vi "Volt2Photon.vi"() -> ()   [LabVIEW 2019]
panel:
  out "Actual Output (V)":dbl format="%#_6p"
  in  "Lockin Sensitivity":dbl format="%#_3p"
  in  "Lockin Output (V)":dbl format="%#_3p"
  out "Mean Power (W)":dbl=-4.8720373573303983e-11 format="%#.3p"
  out "Photons/Pulse":ext=-1.22632021926945247725 format="%#.4g"
  in  "Repetition Rate (Hz)":ext[unit]=80000000.0 format="%#_6p"
  in  "Wavelength (m)":dbl=4e-07 format="%#_6p"
  out "Photons/Second":ext[unit]=-98105617.54155619818 format="%#.0p"
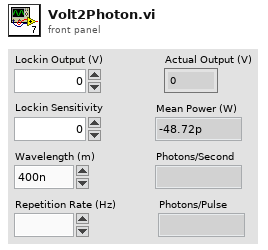
[diagram p1: front panel]
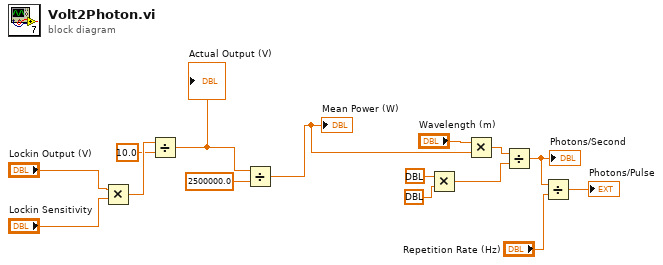
[diagram p0: block diagram]
diagram:
  n1 = Multiply(x="Lockin Output (V)", y="Lockin Sensitivity") -> (x*y=w3:dbl)
  n2 = Divide(x=w3, y=10.0) -> (x/y=w1:dbl)
  "Actual Output (V)" <- w1
  n3 = Divide(x=w1, y=2500000.0) -> (x/y=w6:dbl)
  "Mean Power (W)" <- w6
  n4 = Multiply(x=ext[unit] 6.62607004e-34, y=ext[unit] 299792458.0) -> (x*y=w14:ext[unit])
  n5 = Multiply(x="Wavelength (m)", y=w6) -> (x*y=w13:dbl)
  n6 = Divide(x=w13, y=w14) -> (x/y=w8:ext[unit])
  "Photons/Second" <- w8
  n7 = Divide(x=w8, y="Repetition Rate (Hz)") -> (x/y=→"Photons/Pulse":ext)
